vi "StandAloneTransient_SingleGraphCreation_DataCollection_Light.vi"(9 "wfm":i16[][](array[numeric]), 10 "index":i32, 11 "wfm info":T1(array[cluster])) -> (3 "Array":dbl[](array[numeric]))   [LabVIEW 2019]
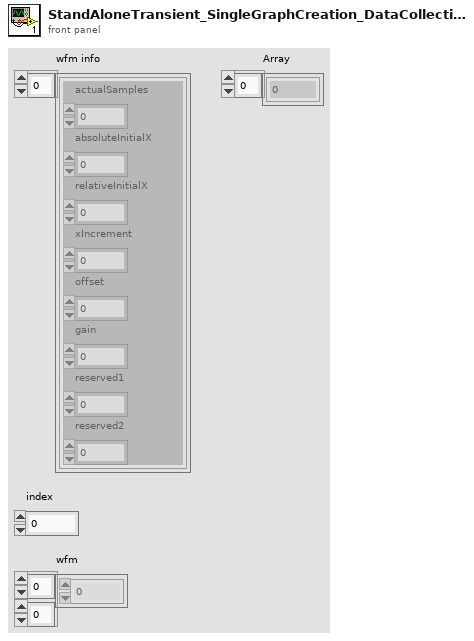
[diagram p1: front panel]
types:
  T1 = cluster{"actualSamples":i32, "absoluteInitialX":dbl, "relativeInitialX":dbl, "xIncrement":dbl, "offset":dbl, "gain":dbl, "reserved1":dbl, "reserved2":dbl}[]
  T2 = cluster{"actualSamples":i32, "absoluteInitialX":dbl, "relativeInitialX":dbl, "xIncrement":dbl, "offset":dbl, "gain":dbl, "reserved1":dbl, "reserved2":dbl}
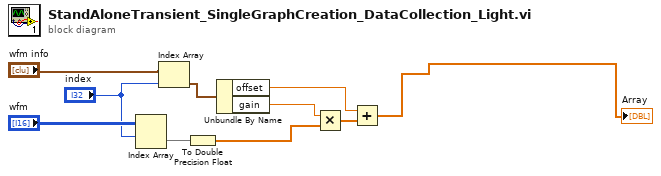
[diagram p0: block diagram]
diagram:
  n1 = Index Array(array="wfm", index (row)="index") -> (element=w6:i16[])  [unwired: 1 in]
  n2 = Index Array(array="wfm info", index="index") -> (element=w5:T2)
  n3 = To Double Precision Float(number=w6) -> (double precision float=w10:dbl[])
  n4 = Unbundle By Name(w5) -> ("offset"=w8:dbl, "gain"=w9:dbl)
  n5 = Multiply(x=w9, y=w10) -> (x*y=w7:dbl[])
  n6 = Add(x=w8, y=w7) -> (x+y=→"Array":dbl[])
